vi "GLOBAL_PedCals_Dig1.vi"(9 "State":enum16{"Initialise", "Write", "Read"}(ring), 10 "Data In":dbl[][](array[numeric])) -> (2 "Data Out":dbl[][](array[numeric]))   [LabVIEW 2014]
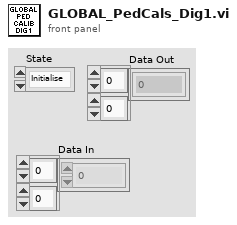
[diagram p1: front panel]
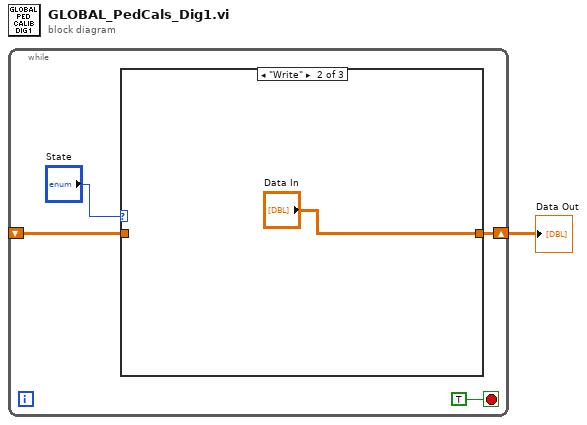
[diagram p0: block diagram]
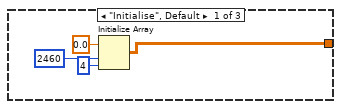
[diagram p2: hidden frame]
diagram:
  n1 = while {
    shift-right: [w3] -> w1
    shift-left: _ -> [w2]
    stop <- TRUE stop-if-true
    n2 = case shown="\"Write\"" "State" {
      tunnel: [w7 "Data In" w11] -> w3
      tunnel: w2 -> [_ _ w11]
      frame "Initialise", Default {
        n3 = Initialize Array(0.0 ("element"), 2460 ("dimension size"), 4 ("dimension size")) -> (w7:dbl[][])
      }
      frame "Write" {
      }
      frame "Read" {
      }
    }
  }
  "Data Out" <- w1
